vi "GV pixelclock.vi"() -> ()   [LabVIEW 2017]
panel:
  out "Pixelclock":bool
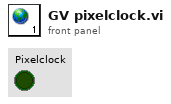
[diagram p1: front panel]
diagram:
